vi "SharedNOM.vi"(1 "Write?":bool, 2 "NumberOfMotorsInput":i32) -> (0 "NumberOfMotors":i32)   [LabVIEW 2010, in "Player.lvlib"]
uses:
  Player.lvlib
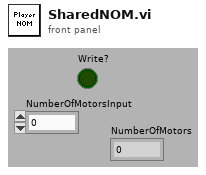
[diagram p1: front panel]
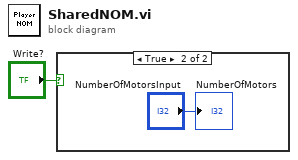
[diagram p0: block diagram]
diagram:
  n1 = case shown="True" "Write?" {
    frame False {
    }
    frame True {
      "NumberOfMotors" <- "NumberOfMotorsInput"
    }
  }
